vi "sub_main_timer.vi"(8 "error in":errorcluster) -> (0 "error out":errorcluster)   [LabVIEW 2019]
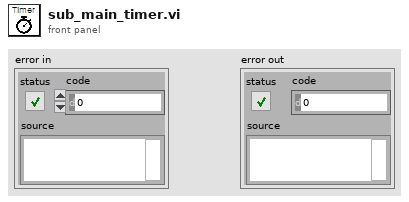
[diagram p1: front panel]
types:
  T1 = typedef "state.ctl" = enum16{"init", "Test circular track", "start point", "start heading adjust", "wait before start", "stop point check", "stop point start", "end point", "entering ending point", "move", "move heading adjust"}
  T2 = cluster{"total time":dbl, "run time":dbl, "pause time":dbl}
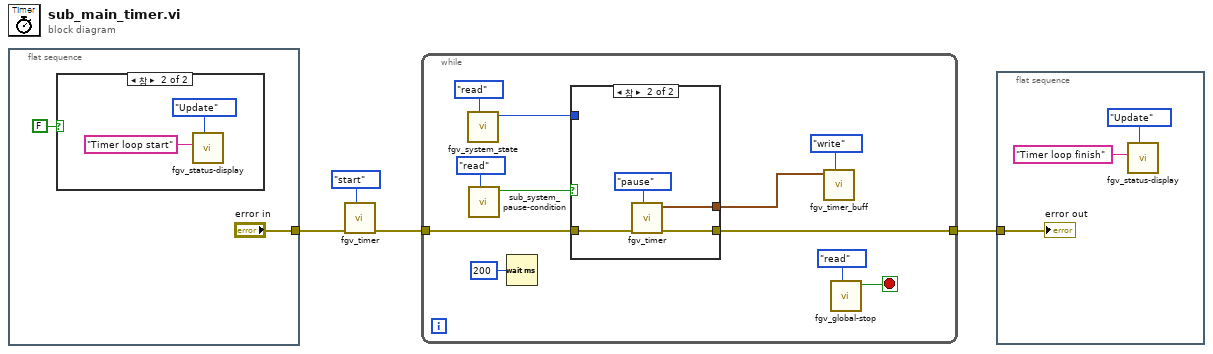
[diagram p0: block diagram]
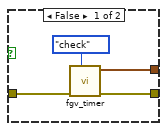
[diagram p3: hidden frame]
diagram:
  n1 = flat-sequence {
    tunnel: ["error in"] -> w4
    frame #0 {
      n2 = case shown="참" FALSE {
        frame False {
        }
        frame True {
          n3 = call "fgv_status-display.vi"("Mode"=enum16{"Initial", "Update", "Clear"}."Update", "title"="Timer loop start" ("String in 1")) -> ()  [unwired: 9 in, 1 out]
        }
      }
    }
  }
  n4 = call "fgv_timer.vi"("cmd"=enum16{"check", "start", "pause"}."start", "error in"=w4) -> ("error out"=w3:errorcluster)  [unwired: 7 in, 2 out]
  n5 = while {
    tunnel: w3 -> [w19]
    tunnel: [w13] -> w1
    stop <- w9 stop-if-true
    n6 = call "fgv_system_state.vi"("cmd"=enum16{"init", "read", "write"}."read") -> ("State out"=w14:T1)  [unwired: 9 in, 1 out]
    n7 = call "sub_system_pause-condition.vi"("cmd"=enum16{"pause", "go", "read"}."read") -> ("pause"=w18:bool)  [unwired: 10 in]
    n8 = Wait (ms)(milliseconds to wait=u32 200) -> ()  [unwired: 1 out]
    n9 = case shown="참" w18 {
      tunnel: w19 -> [w23 w26]
      tunnel: w14 -> [_ _]
      tunnel: [w21 w25] -> w13
      tunnel: [w22 w24] -> w12
      frame False {
        n10 = call "fgv_timer.vi"("cmd"=enum16{"check", "start", "pause"}."check", "error in"=w23) -> ("error out"=w21:errorcluster, "time_status_out"=w22:T2)  [unwired: 7 in, 1 out]
      }
      frame True {
        n11 = call "fgv_timer.vi"("cmd"=enum16{"check", "start", "pause"}."pause", "error in"=w26) -> ("error out"=w25:errorcluster, "time_status_out"=w24:T2)  [unwired: 7 in, 1 out]
      }
    }
    n12 = call "fgv_timer_buff.vi"("cmd"=enum16{"write", "read"}."write", "time_status in"=w12) -> ()  [unwired: 9 in, 1 out]
    n13 = call "fgv_global-stop.vi"("cmd"=enum16{"init", "stop", "read"}."read") -> ("val_out"=w9:bool)  [unwired: 10 in]
  }
  n14 = flat-sequence {
    tunnel: w1 -> [w30]
    frame #0 {
      n15 = call "fgv_status-display.vi"("Mode"=enum16{"Initial", "Update", "Clear"}."Update", "title"="Timer loop finish" ("String in 1")) -> ()  [unwired: 9 in, 1 out]
      "error out" <- w30
    }
  }
